vi "Create_Trajectory_Value_Inches_To_Units.vi"(6 "Units Selector":T1, 11 "Inches":dbl) -> (3 "Units":dbl)   [LabVIEW 2019]
doc: "Convert given units to Meter"
uses:
  CreateTrajectoryENUM/TrajCreateUnitsENUM.ctl
  <vilib>/Rock Robotics/WPI/ThirdParty/JAS_Junk/TrajLib/Trajectory_Library.lvlib
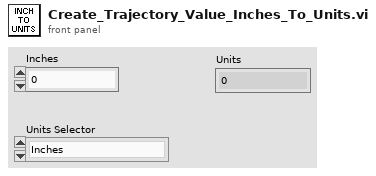
[diagram p1: front panel]
types:
  T1 = typedef "TrajCreateUnitsENUM.ctl" = enum16{"Inches", "Feet", "Centimeters", "Meters"}
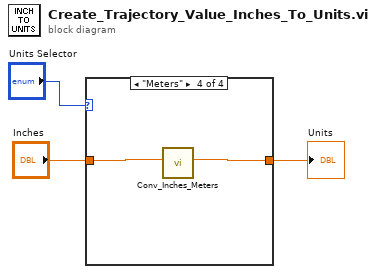
[diagram p0: block diagram]
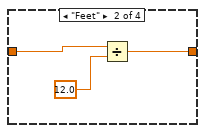
[diagram p3: hidden frame]
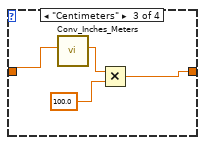
[diagram p4: hidden frame]
diagram:
  n1 = case shown="\"Meters\"" "Units Selector" {
    tunnel: [w4 w7 w10 w12] -> w3
    tunnel: "Inches" -> [w4 w6 w9 w13]
    frame "Inches" {
    }
    frame "Feet" {
      n2 = Divide(x=w6, y=12.0) -> (x/y=w7:dbl)
    }
    frame "Centimeters" {
      n3 = call <vilib>:"Conv_Inches_Meters.vi"("INCH"=w9) -> ("Meters"=w8:dbl)  [unwired: 10 in]
      n4 = Multiply(x=w8, y=100.0) -> (x*y=w10:dbl)
    }
    frame "Meters" {
      n5 = call <vilib>:"Conv_Inches_Meters.vi"("INCH"=w13) -> ("Meters"=w12:dbl)  [unwired: 10 in]
    }
  }
  "Units" <- w3
